vi "DSE7_x_defaut.vi"(2 "tmax":dbl, 3 "Weibull (paramètres)":T2) -> (1 "sér. (s)":T1)   [LabVIEW 2010, in "lv_02.lvlib"]
uses:
  p_5E7_LW.ctl
  lv_01/do_serie-c.ctl
  lv_01/0002-03.vi
  lv_02.lvlib
  lv_01/lv_01.lvlib
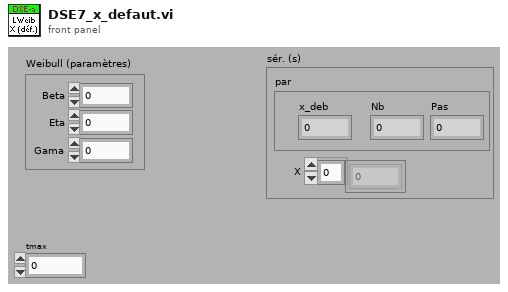
[diagram p1: front panel]
types:
  T1 = typedef "lv_01.lvlib/do_serie-c.ctl" = cluster{"X":dbl[], "par":cluster{"x_deb":dbl, "Pas":dbl, "Nb":dbl}}
  T2 = typedef "lv_02.lvlib/p_5E7_LW.ctl" = cluster{"Beta":dbl, "Eta":dbl, "Gama":dbl}
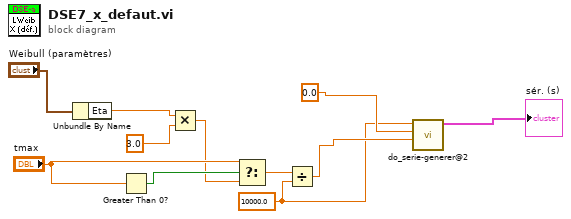
[diagram p0: block diagram]
diagram:
  w1 = 10000.0 ("y")
  n1 = Unbundle By Name("Weibull (paramètres)") -> ("Eta"=w5:dbl)
  n2 = Greater Than 0?(x="tmax") -> (x > 0?=w11:bool)
  n3 = Multiply(x=w5, y=3.0) -> (x*y=w7:dbl)
  n4 = Select(t="tmax", s=w11, f=w7) -> (s? t:f=w9:dbl)
  n5 = Divide(x=w9, y=w1) -> (x/y=w3:dbl)
  n6 = call-poly "do_serie-generer@2.vi"("Pas"=w3, "x_deb"=0.0, "Nb"=w1) -> ("sér. (s)"=→"sér. (s)":T1)  [unwired: 8 in]
